vi "Functional Test Panel.vi"(0 "System#":u8, 7 "Rack Number":i8=1 min=1 max=16, 8 "AutoAge.ini  File Path":path=path "\\\\Beco\\autoage/config/autoage.ini") -> ()   [LabVIEW 2021]
uses:
  Main Controls System v8.0/AutoAge Globals.vi
panel:
  in  "Cancel":bool
  in  "Done":bool
  in  "Update":bool
  in  "Row33 to 40":bool
  in  "Row25 to 32":bool
  in  "Row17 to 24":bool
  in  "Row9 to 16":bool
  in  "Row1 to 8":bool
  in  "Select All":bool
  in  "40":bool
  in  "39":bool
  in  "38":bool
  in  "37":bool
  in  "36":bool
  in  "35":bool
  in  "34":bool
  in  "33":bool
  in  "32":bool
  in  "31":bool
  in  "30":bool
  in  "29":bool
  in  "28":bool
  in  "27":bool
  in  "26":bool
  in  "25":bool
  in  "24":bool
  in  "23":bool
  in  "22":bool
  in  "21":bool
  in  "20":bool
  in  "19":bool
  in  "18":bool
  in  "17":bool
  in  "16":bool
  in  "15":bool
  in  "14":bool
  in  "13":bool
  in  "12":bool
  in  "11":bool
  in  "10":bool
  in  "9":bool
  in  "8":bool
  in  "7":bool
  in  "6":bool
  in  "5":bool
  in  "4":bool
  in  "3":bool
  in  "2":bool
  in  "1":bool
  out "Rack":i8=1 min=1 max=16
  # "Click to turn on the inactive positions.  A red square   in a position indicates that a position is going to run."
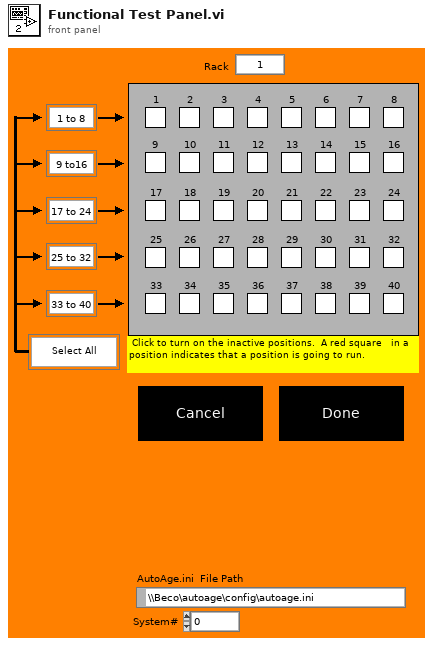
[diagram p1: front panel]
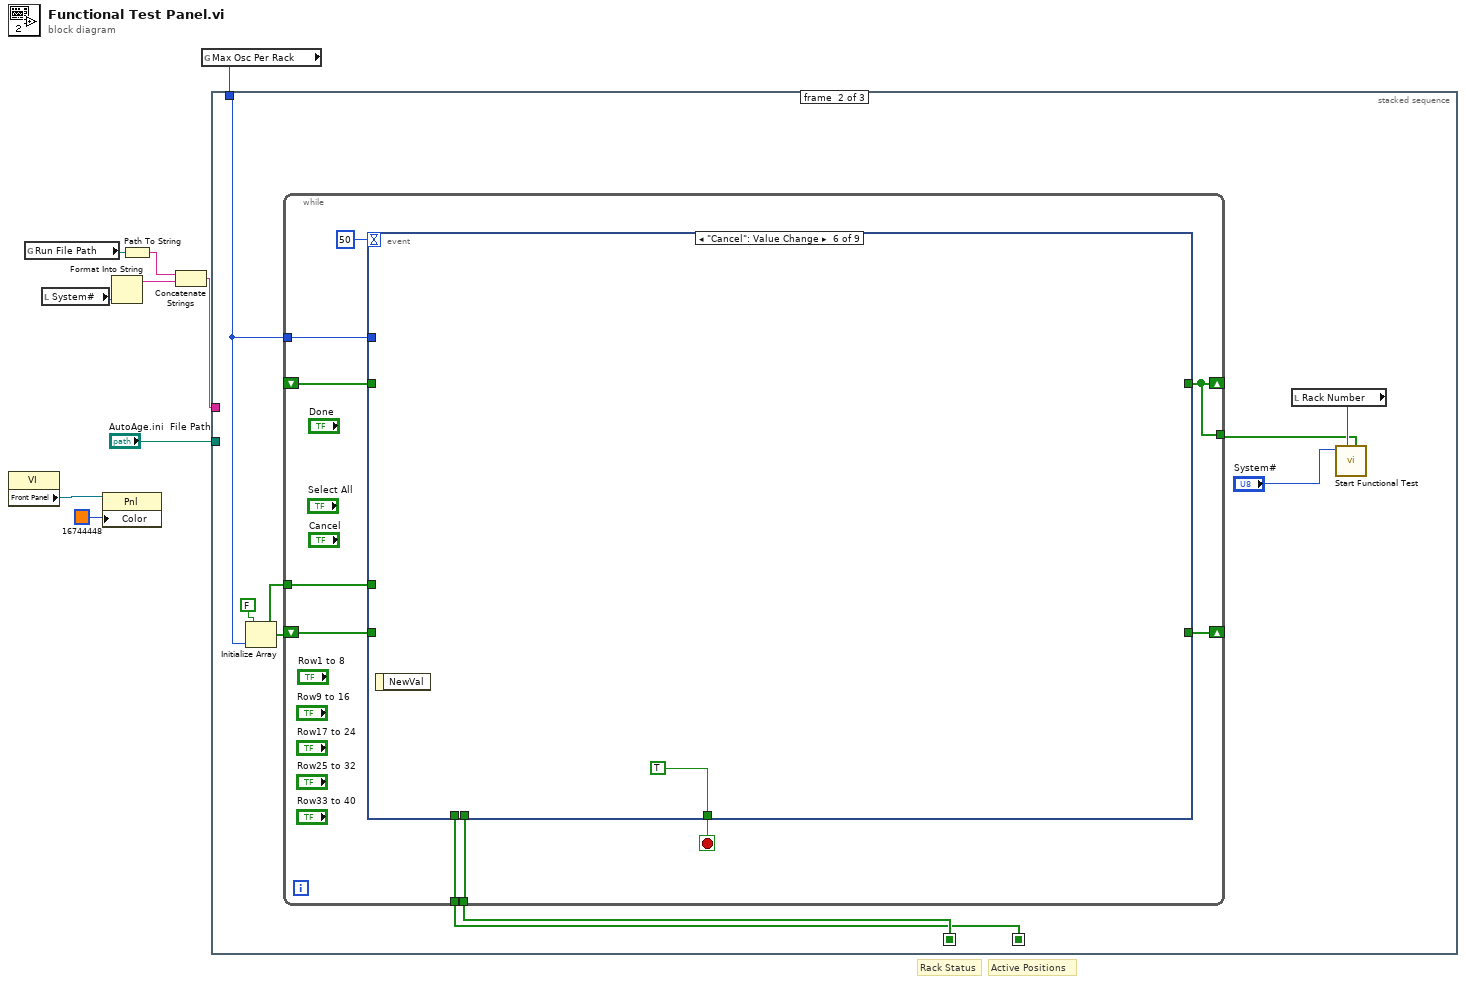
[diagram p0: block diagram]
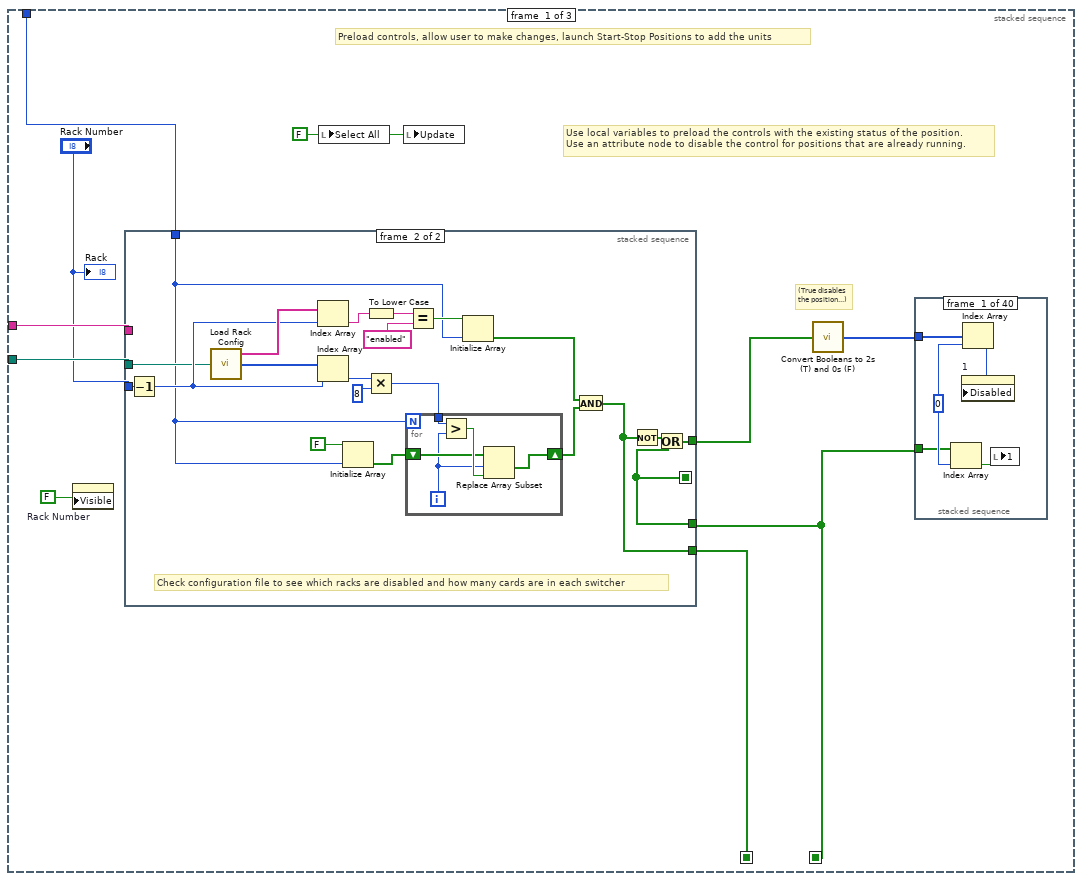
[diagram p2: hidden frame]
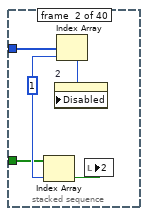
[diagram p3: hidden frame]
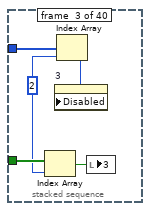
[diagram p4: hidden frame]
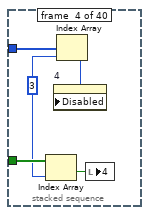
[diagram p5: hidden frame]
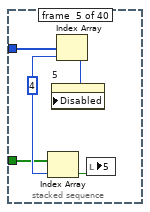
[diagram p6: hidden frame]
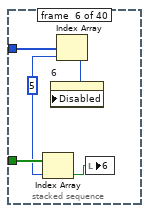
[diagram p7: hidden frame]
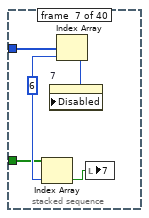
[diagram p8: hidden frame]
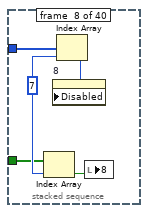
[diagram p9: hidden frame]
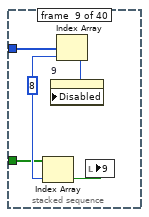
[diagram p10: hidden frame]
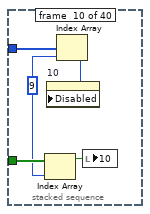
[diagram p11: hidden frame]
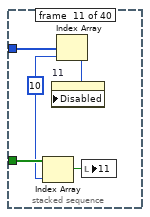
[diagram p12: hidden frame]
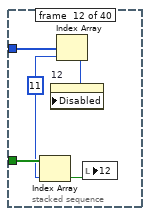
[diagram p13: hidden frame]
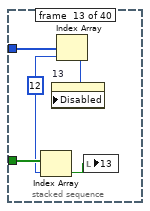
[diagram p14: hidden frame]
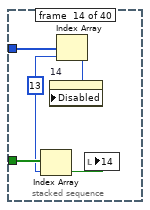
[diagram p15: hidden frame]
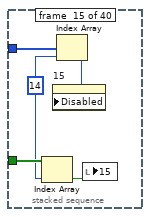
[diagram p16: hidden frame]
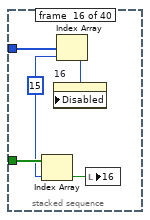
[diagram p17: hidden frame]
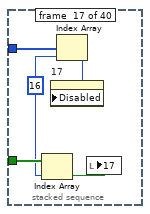
[diagram p18: hidden frame]
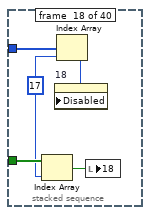
[diagram p19: hidden frame]
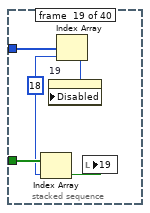
[diagram p20: hidden frame]
diagram:
  # "Active Positions"
  # "Rack Status"
  n1 = property class="VI"() -> ("Front Panel"=w2:refnum<vi>)  [unwired: 2 in, 2 out]
  n2 = global read "AutoAge Globals.vi" "Run File Path"() -> (w8:path)
  n3 = local read "System#"() -> (w7:u8)
  n4 = property class="Pnl"(reference=w2, "Color"=u32 16744448) -> ()  [unwired: 1 in, 2 out]
  n5 = Format Into String(w7) -> (resulting string=w5:string)  [unwired: 3 in, 1 out]
  n6 = Path To String(path=w8) -> (string=w6:string)
  n7 = Concatenate Strings(w6, w5) -> (w4:string)
  n8 = global read "AutoAge Globals.vi" "Max Osc Per Rack"() -> (w3:u16)
  n9 = stacked-sequence {
    seq-local: [w15 _ _] -> [_ w272 _]
    seq-local: [w10 _ _] -> [_ w273 _]
    tunnel: "AutoAge.ini  File Path" -> [w18 _ _]
    tunnel: w4 -> [w17 _ _]
    tunnel: w3 -> [w13 w276 _]
    frame #0 {
      w12 = FALSE ("Select All")
      # "(True disables\nthe position...)"
      # "Preload controls, allow user to make changes, launch Start-Stop Positions to add the units"
      # "Use local variables to preload the controls with the existing status of the position.\nUse an attribute node to disable the control for positions that are already running."
      n10 = property on="Rack Number" class="DigNum (strict)"("Visible"=FALSE) -> ()  [unwired: 2 in, 2 out]
      n11 = stacked-sequence {
        seq-local: [w223 _] -> [_ w249]
        tunnel: "Rack Number" -> [w222 w257]
        tunnel: [_ w248] -> w11
        tunnel: [_ w249] -> w15
        tunnel: w18 -> [_ w246]
        tunnel: w17 -> [w221 _]
        tunnel: w13 -> [w220 w245]
        tunnel: [_ w243] -> w10
        frame #0 {
          # "Scan the disk to see which positions are currently running"
          n12 = for {
            N: w220 -> [_]
            tunnel: [w241] -> w223 mode=indexing
            tunnel: w222 -> [w229]
            tunnel: w221 -> [w226]
            i -> [w242]
            w227 = "-"
            n13 = Increment(x=w242) -> (x+1=w230:i32)
            n14 = Number To Decimal String(number=w229) -> (decimal integer string=w233:string)  [unwired: 1 in]
            n15 = Number To Decimal String(number=w230) -> (decimal integer string=w232:string)  [unwired: 1 in]
            n16 = Concatenate Strings(w226, w227, w233, w227, w232, ".run") -> (w231:string)
            n17 = String To Path(string=w231) -> (path=w240:path)
            n18 = Open/Create/Replace File(file path (use dialog)=w240, access (0:read/write)=1) -> (refnum out=w224:refnum<file>, error out=w225:errorcluster)  [unwired: 4 in, 1 out]
            n19 = Deny Access(4:w225, 6:1, 7:w224) -> (0:w237:errorcluster, 3:w234:refnum<file>)
            n20 = Close File(refnum=w234) -> ()  [unwired: 1 in, 2 out]
            n21 = Unbundle(w237) -> ("code"=w235:i32)  [unwired: 2 out]
            n22 = Equal?(x=w235, y=0) -> (x = y?=w241:bool)
          }
        }
        frame #1 {
          # "Check configuration file to see which racks are disabled and how many cards are in each switcher"
          n23 = Decrement(x=w257) -> (x-1=w247:i8)
          n24 = call "Load Rack Config"("AutoAge.ini  File Path"=w246) -> ("Rack Status"=w258:string[], "# of Cards"=w262:i32[])  [unwired: 1 out]
          n25 = Index Array(array=w258, index=w247) -> (element=w256:string)
          n26 = Index Array(array=w262, index=w247) -> (element=w263:i32)
          n27 = Initialize Array(FALSE, w245) -> (w252:bool[])
          n28 = To Lower Case(string=w256) -> (all lower case string=w261:string)
          n29 = Multiply(x=w263, y=8) -> (x*y=w253:i32)
          n30 = for {
            N: w245 -> [_]
            tunnel: w253 -> [w268]
            shift-right: [w265] -> w250
            shift-left: w252 -> [w266]
            i -> [w264]
            n31 = Greater?(x=w268, y=w264) -> (0:w267:bool)
            n32 = Replace Array Subset(array=w266, new element=w267, index=w264) -> (w265:bool[])
          }
          n33 = Equal?(x=w261, y="enabled") -> (x = y?=w255:bool)
          n34 = Initialize Array(w255, w245) -> (w251:bool[])
          n35 = And(x=w251, y=w250) -> (x .and. y?=w243:bool[])
          n36 = Not(x=w243) -> (.not. x?=w244:bool[])
          n37 = Or(x=w244, y=w249) -> (x .or. y?=w248:bool[])
        }
      }
      n38 = local write "Select All"(w12) -> ()
      n39 = local write "Update"(w12) -> ()
      n40 = call "Convert Booleans to 2s (T) and 0s (F)"("Boolean Array"=w11) -> ("2s and 0s"=w14:u8[])
      n41 = stacked-sequence {
        tunnel: w14 -> [w24 w29 w34 w39 w44 w49 w54 w59 w64 w69 w74 w79 w84 w89 w94 w99 w104 w109 w114 w119 w124 w129 w134 w139 w144 w149 w154 w159 w164 w169 w174 w179 w184 w189 w194 w199 w204 w209 w214 w219]
        tunnel: w15 -> [w21 w26 w33 w38 w42 w48 w52 w57 w62 w68 w73 w78 w83 w88 w93 w98 w103 w108 w113 w118 w123 w128 w133 w138 w143 w148 w153 w158 w163 w168 w173 w178 w183 w188 w193 w198 w203 w208 w213 w216]
        frame #0 {
          w22 = 0
          n42 = Index Array(array=w21, index=w22) -> (element=w23:bool)
          n43 = Index Array(array=w24, index=w22) -> (element=w20:u8)
          n44 = property on="1" class="Bool (strict)"("Disabled"=w20) -> ()  [unwired: 2 in, 2 out]
          n45 = local write "1"(w23) -> ()
        }
        frame #1 {
          w28 = 1
          n46 = Index Array(array=w26, index=w28) -> (element=w27:bool)
          n47 = Index Array(array=w29, index=w28) -> (element=w25:u8)
          n48 = property on="2" class="Bool (strict)"("Disabled"=w25) -> ()  [unwired: 2 in, 2 out]
          n49 = local write "2"(w27) -> ()
        }
        frame #2 {
          w32 = 2
          n50 = Index Array(array=w33, index=w32) -> (element=w31:bool)
          n51 = Index Array(array=w34, index=w32) -> (element=w30:u8)
          n52 = property on="3" class="Bool (strict)"("Disabled"=w30) -> ()  [unwired: 2 in, 2 out]
          n53 = local write "3"(w31) -> ()
        }
        frame #3 {
          w37 = 3
          n54 = Index Array(array=w38, index=w37) -> (element=w36:bool)
          n55 = Index Array(array=w39, index=w37) -> (element=w35:u8)
          n56 = property on="4" class="Bool (strict)"("Disabled"=w35) -> ()  [unwired: 2 in, 2 out]
          n57 = local write "4"(w36) -> ()
        }
        frame #4 {
          w43 = 4
          n58 = Index Array(array=w42, index=w43) -> (element=w41:bool)
          n59 = Index Array(array=w44, index=w43) -> (element=w40:u8)
          n60 = property on="5" class="Bool (strict)"("Disabled"=w40) -> ()  [unwired: 2 in, 2 out]
          n61 = local write "5"(w41) -> ()
        }
        frame #5 {
          w47 = 5
          n62 = Index Array(array=w48, index=w47) -> (element=w46:bool)
          n63 = Index Array(array=w49, index=w47) -> (element=w45:u8)
          n64 = property on="6" class="Bool (strict)"("Disabled"=w45) -> ()  [unwired: 2 in, 2 out]
          n65 = local write "6"(w46) -> ()
        }
        frame #6 {
          w53 = 6
          n66 = Index Array(array=w52, index=w53) -> (element=w51:bool)
          n67 = Index Array(array=w54, index=w53) -> (element=w50:u8)
          n68 = property on="7" class="Bool (strict)"("Disabled"=w50) -> ()  [unwired: 2 in, 2 out]
          n69 = local write "7"(w51) -> ()
        }
        frame #7 {
          w58 = 7
          n70 = Index Array(array=w57, index=w58) -> (element=w56:bool)
          n71 = Index Array(array=w59, index=w58) -> (element=w55:u8)
          n72 = property on="8" class="Bool (strict)"("Disabled"=w55) -> ()  [unwired: 2 in, 2 out]
          n73 = local write "8"(w56) -> ()
        }
        frame #8 {
          w63 = 8
          n74 = Index Array(array=w62, index=w63) -> (element=w61:bool)
          n75 = Index Array(array=w64, index=w63) -> (element=w60:u8)
          n76 = property on="9" class="Bool (strict)"("Disabled"=w60) -> ()  [unwired: 2 in, 2 out]
          n77 = local write "9"(w61) -> ()
        }
        frame #9 {
          w66 = 9
          n78 = Index Array(array=w68, index=w66) -> (element=w67:bool)
          n79 = Index Array(array=w69, index=w66) -> (element=w65:u8)
          n80 = property on="10" class="Bool (strict)"("Disabled"=w65) -> ()  [unwired: 2 in, 2 out]
          n81 = local write "10"(w67) -> ()
        }
        frame #10 {
          w71 = 10
          n82 = Index Array(array=w73, index=w71) -> (element=w72:bool)
          n83 = Index Array(array=w74, index=w71) -> (element=w70:u8)
          n84 = property on="11" class="Bool (strict)"("Disabled"=w70) -> ()  [unwired: 2 in, 2 out]
          n85 = local write "11"(w72) -> ()
        }
        frame #11 {
          w76 = 11
          n86 = Index Array(array=w78, index=w76) -> (element=w77:bool)
          n87 = Index Array(array=w79, index=w76) -> (element=w75:u8)
          n88 = property on="12" class="Bool (strict)"("Disabled"=w75) -> ()  [unwired: 2 in, 2 out]
          n89 = local write "12"(w77) -> ()
        }
        frame #12 {
          w81 = 12
          n90 = Index Array(array=w83, index=w81) -> (element=w82:bool)
          n91 = Index Array(array=w84, index=w81) -> (element=w80:u8)
          n92 = property on="13" class="Bool (strict)"("Disabled"=w80) -> ()  [unwired: 2 in, 2 out]
          n93 = local write "13"(w82) -> ()
        }
        frame #13 {
          w87 = 13
          n94 = Index Array(array=w88, index=w87) -> (element=w86:bool)
          n95 = Index Array(array=w89, index=w87) -> (element=w85:u8)
          n96 = property on="14" class="Bool (strict)"("Disabled"=w85) -> ()  [unwired: 2 in, 2 out]
          n97 = local write "14"(w86) -> ()
        }
        frame #14 {
          w92 = 14
          n98 = Index Array(array=w93, index=w92) -> (element=w91:bool)
          n99 = Index Array(array=w94, index=w92) -> (element=w90:u8)
          n100 = property on="15" class="Bool (strict)"("Disabled"=w90) -> ()  [unwired: 2 in, 2 out]
          n101 = local write "15"(w91) -> ()
        }
        frame #15 {
          w97 = 15
          n102 = Index Array(array=w98, index=w97) -> (element=w96:bool)
          n103 = Index Array(array=w99, index=w97) -> (element=w95:u8)
          n104 = property on="16" class="Bool (strict)"("Disabled"=w95) -> ()  [unwired: 2 in, 2 out]
          n105 = local write "16"(w96) -> ()
        }
        frame #16 {
          w102 = 16
          n106 = Index Array(array=w103, index=w102) -> (element=w101:bool)
          n107 = Index Array(array=w104, index=w102) -> (element=w100:u8)
          n108 = property on="17" class="Bool (strict)"("Disabled"=w100) -> ()  [unwired: 2 in, 2 out]
          n109 = local write "17"(w101) -> ()
        }
        frame #17 {
          w107 = 17
          n110 = Index Array(array=w108, index=w107) -> (element=w106:bool)
          n111 = Index Array(array=w109, index=w107) -> (element=w105:u8)
          n112 = property on="18" class="Bool (strict)"("Disabled"=w105) -> ()  [unwired: 2 in, 2 out]
          n113 = local write "18"(w106) -> ()
        }
        frame #18 {
          w112 = 18
          n114 = Index Array(array=w113, index=w112) -> (element=w111:bool)
          n115 = Index Array(array=w114, index=w112) -> (element=w110:u8)
          n116 = property on="19" class="Bool (strict)"("Disabled"=w110) -> ()  [unwired: 2 in, 2 out]
          n117 = local write "19"(w111) -> ()
        }
        frame #19 {
          w117 = 19
          n118 = Index Array(array=w118, index=w117) -> (element=w116:bool)
          n119 = Index Array(array=w119, index=w117) -> (element=w115:u8)
          n120 = property on="20" class="Bool (strict)"("Disabled"=w115) -> ()  [unwired: 2 in, 2 out]
          n121 = local write "20"(w116) -> ()
        }
        frame #20 {
          w121 = 20
          n122 = Index Array(array=w123, index=w121) -> (element=w122:bool)
          n123 = Index Array(array=w124, index=w121) -> (element=w120:u8)
          n124 = property on="21" class="Bool (strict)"("Disabled"=w120) -> ()  [unwired: 2 in, 2 out]
          n125 = local write "21"(w122) -> ()
        }
        frame #21 {
          w127 = 21
          n126 = Index Array(array=w128, index=w127) -> (element=w126:bool)
          n127 = Index Array(array=w129, index=w127) -> (element=w125:u8)
          n128 = property on="22" class="Bool (strict)"("Disabled"=w125) -> ()  [unwired: 2 in, 2 out]
          n129 = local write "22"(w126) -> ()
        }
        frame #22 {
          w132 = 22
          n130 = Index Array(array=w133, index=w132) -> (element=w131:bool)
          n131 = Index Array(array=w134, index=w132) -> (element=w130:u8)
          n132 = property on="23" class="Bool (strict)"("Disabled"=w130) -> ()  [unwired: 2 in, 2 out]
          n133 = local write "23"(w131) -> ()
        }
        frame #23 {
          w137 = 23
          n134 = Index Array(array=w138, index=w137) -> (element=w136:bool)
          n135 = Index Array(array=w139, index=w137) -> (element=w135:u8)
          n136 = property on="24" class="Bool (strict)"("Disabled"=w135) -> ()  [unwired: 2 in, 2 out]
          n137 = local write "24"(w136) -> ()
        }
        frame #24 {
          w142 = 24
          n138 = Index Array(array=w143, index=w142) -> (element=w141:bool)
          n139 = Index Array(array=w144, index=w142) -> (element=w140:u8)
          n140 = property on="25" class="Bool (strict)"("Disabled"=w140) -> ()  [unwired: 2 in, 2 out]
          n141 = local write "25"(w141) -> ()
        }
        frame #25 {
          w147 = 25
          n142 = Index Array(array=w148, index=w147) -> (element=w146:bool)
          n143 = Index Array(array=w149, index=w147) -> (element=w145:u8)
          n144 = property on="26" class="Bool (strict)"("Disabled"=w145) -> ()  [unwired: 2 in, 2 out]
          n145 = local write "26"(w146) -> ()
        }
        frame #26 {
          w152 = 26
          n146 = Index Array(array=w153, index=w152) -> (element=w151:bool)
          n147 = Index Array(array=w154, index=w152) -> (element=w150:u8)
          n148 = property on="27" class="Bool (strict)"("Disabled"=w150) -> ()  [unwired: 2 in, 2 out]
          n149 = local write "27"(w151) -> ()
        }
        frame #27 {
          w157 = 27
          n150 = Index Array(array=w158, index=w157) -> (element=w156:bool)
          n151 = Index Array(array=w159, index=w157) -> (element=w155:u8)
          n152 = property on="28" class="Bool (strict)"("Disabled"=w155) -> ()  [unwired: 2 in, 2 out]
          n153 = local write "28"(w156) -> ()
        }
        frame #28 {
          w162 = 28
          n154 = Index Array(array=w163, index=w162) -> (element=w161:bool)
          n155 = Index Array(array=w164, index=w162) -> (element=w160:u8)
          n156 = property on="29" class="Bool (strict)"("Disabled"=w160) -> ()  [unwired: 2 in, 2 out]
          n157 = local write "29"(w161) -> ()
        }
        frame #29 {
          w167 = 29
          n158 = Index Array(array=w168, index=w167) -> (element=w166:bool)
          n159 = Index Array(array=w169, index=w167) -> (element=w165:u8)
          n160 = property on="30" class="Bool (strict)"("Disabled"=w165) -> ()  [unwired: 2 in, 2 out]
          n161 = local write "30"(w166) -> ()
        }
        frame #30 {
          w172 = 30
          n162 = Index Array(array=w173, index=w172) -> (element=w171:bool)
          n163 = Index Array(array=w174, index=w172) -> (element=w170:u8)
          n164 = property on="31" class="Bool (strict)"("Disabled"=w170) -> ()  [unwired: 2 in, 2 out]
          n165 = local write "31"(w171) -> ()
        }
        frame #31 {
          w177 = 31
          n166 = Index Array(array=w178, index=w177) -> (element=w176:bool)
          n167 = Index Array(array=w179, index=w177) -> (element=w175:u8)
          n168 = property on="32" class="Bool (strict)"("Disabled"=w175) -> ()  [unwired: 2 in, 2 out]
          n169 = local write "32"(w176) -> ()
        }
        frame #32 {
          w182 = 32
          n170 = Index Array(array=w183, index=w182) -> (element=w181:bool)
          n171 = Index Array(array=w184, index=w182) -> (element=w180:u8)
          n172 = property on="33" class="Bool (strict)"("Disabled"=w180) -> ()  [unwired: 2 in, 2 out]
          n173 = local write "33"(w181) -> ()
        }
        frame #33 {
          w187 = 33
          n174 = Index Array(array=w188, index=w187) -> (element=w186:bool)
          n175 = Index Array(array=w189, index=w187) -> (element=w185:u8)
          n176 = property on="34" class="Bool (strict)"("Disabled"=w185) -> ()  [unwired: 2 in, 2 out]
          n177 = local write "34"(w186) -> ()
        }
        frame #34 {
          w192 = 34
          n178 = Index Array(array=w193, index=w192) -> (element=w191:bool)
          n179 = Index Array(array=w194, index=w192) -> (element=w190:u8)
          n180 = property on="35" class="Bool (strict)"("Disabled"=w190) -> ()  [unwired: 2 in, 2 out]
          n181 = local write "35"(w191) -> ()
        }
        frame #35 {
          w197 = 35
          n182 = Index Array(array=w198, index=w197) -> (element=w196:bool)
          n183 = Index Array(array=w199, index=w197) -> (element=w195:u8)
          n184 = property on="36" class="Bool (strict)"("Disabled"=w195) -> ()  [unwired: 2 in, 2 out]
          n185 = local write "36"(w196) -> ()
        }
        frame #36 {
          w202 = 36
          n186 = Index Array(array=w203, index=w202) -> (element=w201:bool)
          n187 = Index Array(array=w204, index=w202) -> (element=w200:u8)
          n188 = property on="37" class="Bool (strict)"("Disabled"=w200) -> ()  [unwired: 2 in, 2 out]
          n189 = local write "37"(w201) -> ()
        }
        frame #37 {
          w207 = 37
          n190 = Index Array(array=w208, index=w207) -> (element=w206:bool)
          n191 = Index Array(array=w209, index=w207) -> (element=w205:u8)
          n192 = property on="38" class="Bool (strict)"("Disabled"=w205) -> ()  [unwired: 2 in, 2 out]
          n193 = local write "38"(w206) -> ()
        }
        frame #38 {
          w212 = 38
          n194 = Index Array(array=w213, index=w212) -> (element=w211:bool)
          n195 = Index Array(array=w214, index=w212) -> (element=w210:u8)
          n196 = property on="39" class="Bool (strict)"("Disabled"=w210) -> ()  [unwired: 2 in, 2 out]
          n197 = local write "39"(w211) -> ()
        }
        frame #39 {
          w217 = 39
          n198 = Index Array(array=w216, index=w217) -> (element=w218:bool)
          n199 = Index Array(array=w219, index=w217) -> (element=w215:u8)
          n200 = property on="40" class="Bool (strict)"("Disabled"=w215) -> ()  [unwired: 2 in, 2 out]
          n201 = local write "40"(w218) -> ()
        }
      }
      "Rack" <- "Rack Number"
    }
    frame #1 {
      n202 = Initialize Array(FALSE, w276) -> (w274:bool[])
      n203 = while {
        tunnel: [w283] -> w269
        tunnel: w276 -> [w284]
        tunnel: w273 -> [w285]
        shift-right: [w283] -> _
        shift-left: _ -> [w282]
        shift-right: [w279] -> _
        shift-left: w274 -> [w281]
        tunnel: w274 -> [w280]
        tunnel: w272 -> [w278]
        stop <- w277 stop-if-true
        n204 = event shown="[5] \"Cancel\": Value Change" {
          selector: _ -> [_ _ _ _ _ _ _ _ _]
          dyn-events: _ -> [_ _ _ _ _ _ _ _ _]
          timeout: 50 -> [_ _ _ _ _ _ _ _ _]
          tunnel: [w288 w394 _ _ _ _ _ _ w459] -> w283
          tunnel: w285 -> [w291 _ w401 w412 w423 _ w435 w446 _]
          tunnel: w284 -> [w289 w388 _ _ _ _ _ _ _]
          tunnel: [FALSE FALSE FALSE ("NewVal") FALSE ("NewVal") FALSE ("NewVal") TRUE FALSE FALSE w457] -> w277
          tunnel: w282 -> [_ w394 _ _ _ _ _ _ w459]
          tunnel: w281 -> [w290 w393 w406 w416 w427 _ w440 w451 w458]
          tunnel: w280 -> [_ w392 _ _ _ _ _ _ _]
          tunnel: [w288 w389 w402 w415 w426 _ w439 w450 w458] -> w279
          tunnel: w278 -> [w287 w387 _ _ _ _ _ _ _]
          event Timeout {
            n205 = event-data() -> ()  [unwired: 1 in, 1 out]
            n206 = case shown="True" "Update" {
              tunnel: [w334 w337] -> w288
              tunnel: w291 -> [_ w340]
              tunnel: w290 -> [_ w339]
              tunnel: w289 -> [_ w338]
              tunnel: w287 -> [_ w335]
              frame False {
                # "The actual controls"
                n207 = Build Array("1", "2", "3", "4", "5", "6", "7", "8", "9", "10", "11", "12", "13", "14", "15", "16", "17", "18", "19", "20", "21", "22", "23", "24", "25", "26", "27", "28", "29", "30", "31", "32", "33", "34", "35", "36", "37", "38", "39", "40") -> (w334:bool[])
              }
              frame True {
                # "Update the Control Status"
                n208 = for {
                  N: w338 -> [_]
                  tunnel: w340 -> [w345] mode=indexing
                  tunnel: w339 -> [w344] mode=indexing
                  tunnel: [w342] -> w337 mode=indexing
                  tunnel: w335 -> [w341] mode=indexing
                  i -> [w346]
                  n209 = And(x=w345, y=w344) -> (x .and. y?=w343:bool)
                  n210 = Or(x=w341, y=w343) -> (x .or. y?=w342:bool)
                  n211 = case shown="7" w346 {
                    tunnel: w342 -> [w347 w348 w349 w350 w351 w352 w353 w354 w355 w356 w357 w358 w359 w360 w361 w362 w363 w364 w365 w366 w367 w368 w369 w370 w371 w372 w373 w374 w375 w376 w377 w378 w379 w380 w381 w382 w383 w384 w385 w386]
                    frame 0, Default {
                      n212 = local write "1"(w347) -> ()
                    }
                    frame 1 {
                      n213 = local write "2"(w348) -> ()
                    }
                    frame 2 {
                      n214 = local write "3"(w349) -> ()
                    }
                    frame 3 {
                      n215 = local write "4"(w350) -> ()
                    }
                    frame 4 {
                      n216 = local write "5"(w351) -> ()
                    }
                    frame 5 {
                      n217 = local write "6"(w352) -> ()
                    }
                    frame 6 {
                      n218 = local write "7"(w353) -> ()
                    }
                    frame 7 {
                      n219 = local write "8"(w354) -> ()
                    }
                    frame 8 {
                      n220 = local write "9"(w355) -> ()
                    }
                    frame 9 {
                      n221 = local write "10"(w356) -> ()
                    }
                    frame 10 {
                      n222 = local write "11"(w357) -> ()
                    }
                    frame 11 {
                      n223 = local write "12"(w358) -> ()
                    }
                    frame 12 {
                      n224 = local write "13"(w359) -> ()
                    }
                    frame 13 {
                      n225 = local write "14"(w360) -> ()
                    }
                    frame 14 {
                      n226 = local write "15"(w361) -> ()
                    }
                    frame 15 {
                      n227 = local write "16"(w362) -> ()
                    }
                    frame 16 {
                      n228 = local write "17"(w363) -> ()
                    }
                    frame 17 {
                      n229 = local write "18"(w364) -> ()
                    }
                    frame 18 {
                      n230 = local write "19"(w365) -> ()
                    }
                    frame 19 {
                      n231 = local write "20"(w366) -> ()
                    }
                    frame 20 {
                      n232 = local write "21"(w367) -> ()
                    }
                    frame 21 {
                      n233 = local write "22"(w368) -> ()
                    }
                    frame 22 {
                      n234 = local write "23"(w369) -> ()
                    }
                    frame 23 {
                      n235 = local write "24"(w370) -> ()
                    }
                    frame 24 {
                      n236 = local write "25"(w371) -> ()
                    }
                    frame 25 {
                      n237 = local write "26"(w372) -> ()
                    }
                    frame 26 {
                      n238 = local write "27"(w373) -> ()
                    }
                    frame 27 {
                      n239 = local write "28"(w374) -> ()
                    }
                    frame 28 {
                      n240 = local write "29"(w375) -> ()
                    }
                    frame 29 {
                      n241 = local write "30"(w376) -> ()
                    }
                    frame 30 {
                      n242 = local write "31"(w377) -> ()
                    }
                    frame 31 {
                      n243 = local write "32"(w378) -> ()
                    }
                    frame 32 {
                      n244 = local write "33"(w379) -> ()
                    }
                    frame 33 {
                      n245 = local write "34"(w380) -> ()
                    }
                    frame 34 {
                      n246 = local write "35"(w381) -> ()
                    }
                    frame 35 {
                      n247 = local write "36"(w382) -> ()
                    }
                    frame 36 {
                      n248 = local write "37"(w383) -> ()
                    }
                    frame 37 {
                      n249 = local write "38"(w384) -> ()
                    }
                    frame 38 {
                      n250 = local write "39"(w385) -> ()
                    }
                    frame 39 {
                      n251 = local write "40"(w386) -> ()
                    }
                  }
                }
                n252 = local write "Update"(FALSE ("Update")) -> ()
              }
            }
          }
          event "Select All": Value Change {
            n253 = event-data() -> ("NewVal"=w390:bool)  [unwired: 1 in]
            n254 = case shown="True" w390 {
              tunnel: w393 -> [w396 w397]
              tunnel: w392 -> [_ _]
              tunnel: [w396 w400] -> w389
              tunnel: w387 -> [_ w398]
              tunnel: w388 -> [_ w399]
              frame False {
              }
              frame True {
                n255 = call "Select All Status.vi"("Max Positions per Rack"=w399, "Active Positions"=w397, "Rack Status In"=w398) -> ("Rack Status Out"=w400:bool[])
              }
            }
            n256 = local write "Update"(TRUE ("Update")) -> ()
          }
          event "Row1 to 8": Value Change {
            n257 = event-data() -> ("NewVal"=w405:bool)  [unwired: 1 in]
            n258 = case shown="True" w405 {
              tunnel: w406 -> [w407 w411]
              tunnel: [w407 w410] -> w402
              tunnel: w401 -> [_ w408]
              frame False {
              }
              frame True {
                n259 = call "Check Current Row Status.vi"("Row"=1, "Active Positions"=w408, "Rack Status In"=w411) -> ("Rack Status Out"=w410:bool[])
              }
            }
            n260 = local write "Update"(TRUE ("Update")) -> ()
          }
          event "Row9 to 16": Value Change {
            n261 = event-data() -> ("NewVal"=w417:bool)  [unwired: 1 in]
            n262 = case shown="True" w417 {
              tunnel: w416 -> [w418 w422]
              tunnel: [w418 w421] -> w415
              tunnel: w412 -> [_ w419]
              frame False {
              }
              frame True {
                n263 = call "Check Current Row Status.vi"("Row"=2, "Active Positions"=w419, "Rack Status In"=w422) -> ("Rack Status Out"=w421:bool[])
              }
            }
            n264 = local write "Update"(TRUE ("Update")) -> ()
          }
          event "Row17 to 24": Value Change {
            n265 = event-data() -> ("NewVal"=w428:bool)  [unwired: 1 in]
            n266 = case shown="True" w428 {
              tunnel: w427 -> [w429 w433]
              tunnel: [w429 w432] -> w426
              tunnel: w423 -> [_ w430]
              frame False {
              }
              frame True {
                n267 = call "Check Current Row Status.vi"("Row"=3, "Active Positions"=w430, "Rack Status In"=w433) -> ("Rack Status Out"=w432:bool[])
              }
            }
            n268 = local write "Update"(TRUE ("Update")) -> ()
          }
          event "Cancel": Value Change {
            n269 = event-data() -> ()  [unwired: 1 in, 1 out]
          }
          event "Row25 to 32": Value Change {
            n270 = event-data() -> ("NewVal"=w438:bool)  [unwired: 1 in]
            n271 = case shown="True" w438 {
              tunnel: w440 -> [w441 w445]
              tunnel: [w441 w444] -> w439
              tunnel: w435 -> [_ w442]
              frame False {
              }
              frame True {
                n272 = call "Check Current Row Status.vi"("Row"=4, "Active Positions"=w442, "Rack Status In"=w445) -> ("Rack Status Out"=w444:bool[])
              }
            }
            n273 = local write "Update"(TRUE ("Update")) -> ()
          }
          event "Row33 to 40": Value Change {
            n274 = event-data() -> ("NewVal"=w449:bool)  [unwired: 1 in]
            n275 = case shown="True" w449 {
              tunnel: w451 -> [w452 w456]
              tunnel: [w452 w455] -> w450
              tunnel: w446 -> [_ w453]
              frame False {
              }
              frame True {
                n276 = call "Check Current Row Status.vi"("Row"=5, "Active Positions"=w453, "Rack Status In"=w456) -> ("Rack Status Out"=w455:bool[])
              }
            }
            n277 = local write "Update"(TRUE ("Update")) -> ()
          }
          event "Done": Value Change {
            n278 = event-data() -> ("NewVal"=w457:bool)  [unwired: 1 in]
          }
        }
      }
      n279 = local read "Rack Number"() -> (w270:i8)
      n280 = call "Start Functional Test.vi"("New Status of Positions"=w269, "Rack Number"=w270, "System#"="System#") -> ()  [unwired: 9 in]
    }
    frame #2 {
      # "Set \"Functional Test Required\" to TRUE so Data Acquistion will start the Auto Functional Check on the units just added"
      n281 = global write "Globals" "Functional Test Requested"(TRUE ("Functional Test Requested")) -> ()
    }
  }
